vi "SquareWaveDialog.vi"() -> (6 "FreqString":string, 7 "VoltString":string)   [LabVIEW 2011]
panel:
  in  "OK Button":bool
  in  "Voltage":u8(slide) scale=0.0..3.0
  in  "Frequency":u8(slide) scale=0.0..5.0
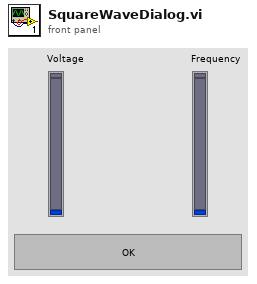
[diagram p1: front panel]
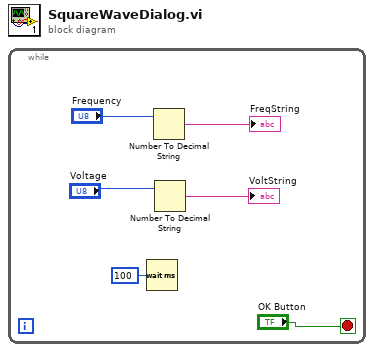
[diagram p0: block diagram]
diagram:
  n1 = while {
    stop <- "OK Button" stop-if-true
    n2 = Wait (ms)(milliseconds to wait=u32 100) -> ()  [unwired: 1 out]
    n3 = Number To Decimal String(number="Frequency") -> (decimal integer string=→"FreqString":string)  [unwired: 1 in]
    n4 = Number To Decimal String(number="Voltage") -> (decimal integer string=→"VoltString":string)  [unwired: 1 in]
  }
